vi "Flock_Server_Build Path to Process.vi"(10 "path":path, 11 "Process":string) -> (3 "Local Process Path":path)   [LabVIEW 2014, in "Flock_Shared_Messaging.lvlib" / "Flock_Shared_CentralProcessMessaging.lvlib"]
uses:
  CentralProcessMessaging/Flock_Shared_CentralProcessMessaging.lvlib
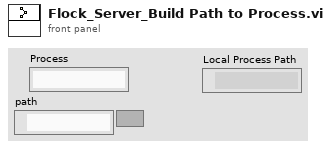
[diagram p1: front panel]
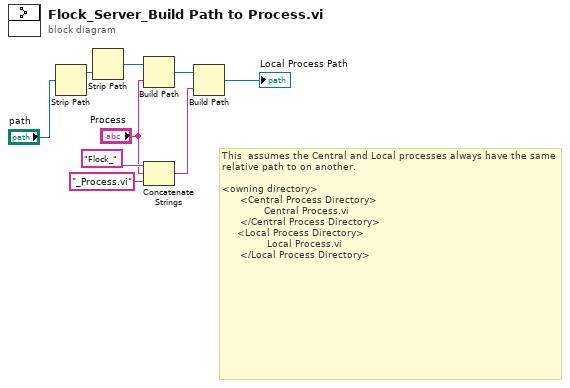
[diagram p0: block diagram]
diagram:
  # "This  assumes the Central and Local processes always have the same relative path to on another. \n\n<owning directory>\n      <Central Process Directory>\n              Central Process.vi\n      </Central Process Directory>\n     <Local Process Directory>\n               Local Process.vi\n      </Local Process Directory>"
  n1 = Strip Path(path="path") -> (stripped path=w3:path)  [unwired: 1 out]
  n2 = Strip Path(path=w3) -> (stripped path=w1:path)  [unwired: 1 out]
  n3 = Build Path(base path=w1, name or relative path="Process") -> (appended path=w8:path)
  n4 = Concatenate Strings("Flock_" ("name or relative path"), "Process", "_Process.vi" ("string")) -> (w4:string)
  n5 = Build Path(base path=w8, name or relative path=w4) -> (appended path=→"Local Process Path":path)
